vi "Discrete PF.vi"   [LabVIEW 2017, in "NI_Gmath.lvlib"]
doc: "Computes the discrete probability function (PF), or the probability that the random variate X, where X describes the selected distribution type, takes on the value <B>n</B>. You must manually select the polymorphic instance to use."
uses:
  <vilib>/gmath/NI_Gmath.lvlib
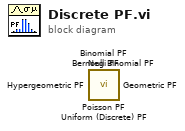
[diagram p0: block diagram]
diagram:
  n1 = call <vilib>:"Poisson PF.vi"() -> ()  [unwired: 10 in, 2 out]
  n2 = call <vilib>:"Neg Binomial PF.vi"() -> ()  [unwired: 10 in, 2 out]
  n3 = call <vilib>:"Hypergeometric PF.vi"() -> ()  [unwired: 10 in, 2 out]
  n4 = call <vilib>:"Geometric PF.vi"() -> ()  [unwired: 10 in, 2 out]
  n5 = call <vilib>:"Uniform (Discrete) PF.vi"() -> ()  [unwired: 10 in, 2 out]
  n6 = call <vilib>:"Binomial PF.vi"() -> ()  [unwired: 10 in, 2 out]
  n7 = call <vilib>:"Bernoulli PF.vi"() -> ()  [unwired: 10 in, 2 out]
